vi "Read RT hardware channels.vi"(8 "error in":errorcluster, 11 "Ballard ARINC-429 Tx Execution Unit in":refnum<class "Ballard ARINC-429 Tx Scheduled Labels Execution Unit.lvclass">) -> (0 "error out":errorcluster, 2 "RT hardware channels":T1[](array[typedef]) {"labels settings for RT"."Label Timestamp Channel Data Reference" format="%.0x"; "labels settings for RT"."Word Initial Raw Value" format="%032.0f"; "labels settings for RT"."Label Disable/Trigger Channel Reference" format="%.0x"; "labels settings for RT"."parameter driver data"."Tx parameter refs" format="%.0x"; "labels settings for RT"."parameter driver data"."Rx block data refs"."Data Reference" format="%.0x"; "labels settings for RT"."SDI" format="%02b"; "labels settings for RT"."label" format="%.0o"}, 3 "Ballard ARINC-429 Tx Execution Unit out":refnum<class "Ballard ARINC-429 Tx Scheduled Labels Execution Unit.lvclass">)   [LabVIEW 2020, in "Ballard ARINC 429 Engine.lvlib" / "Implementation.lvlib" / "Ballard ARINC-429 Tx Scheduled Labels Execution Unit.lvclass"]
uses:
  Ballard ARINC-429 Tx Scheduled Labels Execution Unit.lvclass
  Shared/Label.ctl
  Encoding and Decoding/Encoding.ctl
  Encoding and Decoding/Encoding and Decoding.lvlib
  Shared/Parameter Definition.ctl
  <vilib>/NI VeriStand/Custom Device API/Data Reference.ctl
  <vilib>/NI VeriStand/Custom Device API/Custom Device API.lvlib
  <vilib>/NI VeriStand/Custom Device API/Block Data Reference.ctl
  <vilib>/NI VeriStand/Custom Device API/Custom Device Item Ref.ctl
  Shared/RT Parameters.ctl
  Shared/Transfer Type.ctl
  Shared/RT Label Settings.ctl
  Shared/RT Hardware Channel Settings.ctl
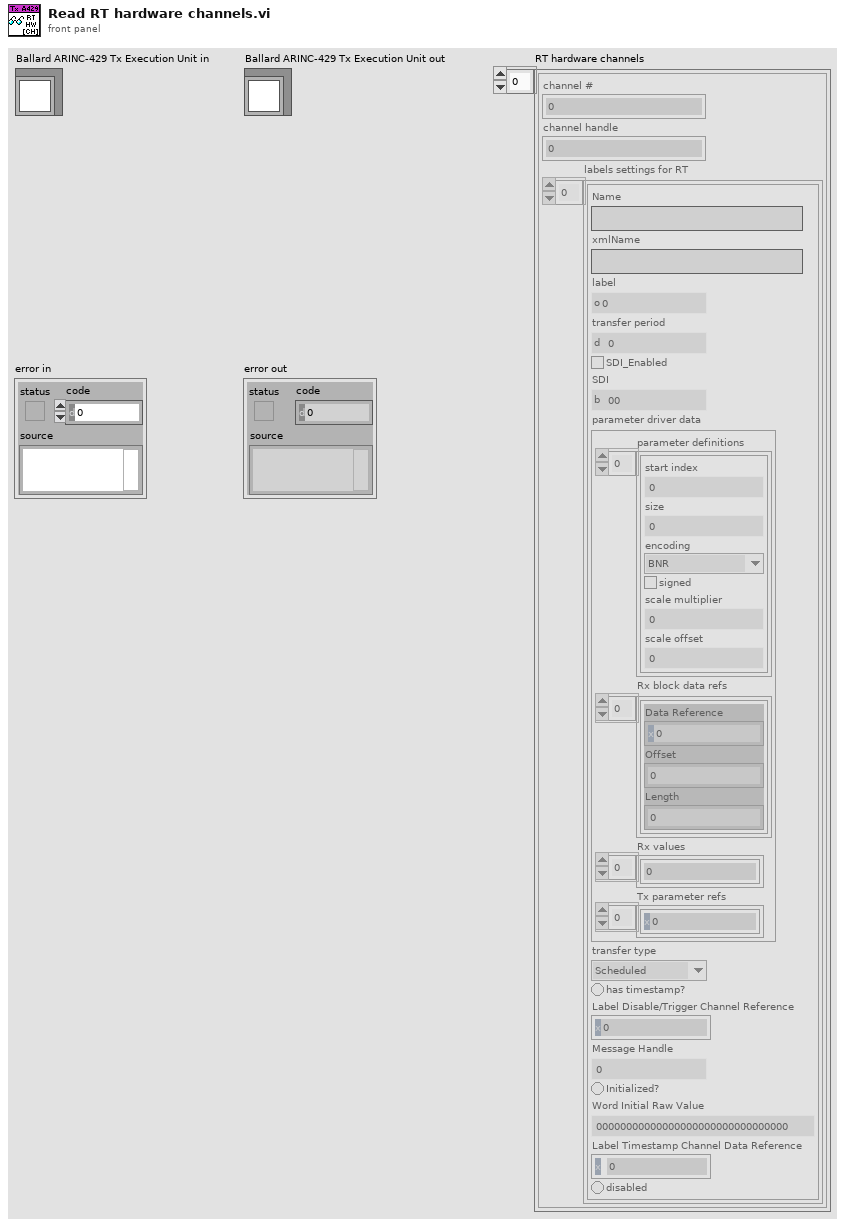
[diagram p1: front panel]
types:
  T1 = typedef "RT Hardware Channel Settings.ctl" = cluster{"channel #":u16, "channel handle":u64, "labels settings for RT":T2[]}
  T2 = typedef "RT Label Settings.ctl" = cluster{"Name":string, "xmlName":string, "label":T3, "transfer period":u32, "SDI_Enabled":bool, "SDI":u8, "parameter driver data":T4, "transfer type":T10, "has timestamp?":bool, "Label Disable/Trigger Channel Reference":T9, "Message Handle":u64, "Initialized?":bool, "Word Initial Raw Value":u32, "Label Timestamp Channel Data Reference":T8, "disabled":bool}
  T3 = typedef "Label.ctl" = u8
  T4 = typedef "RT Parameters.ctl" = cluster{"parameter definitions":T5[], "Rx block data refs":T7[], "Rx values":dbl[], "Tx parameter refs":T9[]}
  T5 = typedef "Parameter Definition.ctl" = cluster{"start index":i32, "size":i32, "encoding":T6, "signed":bool, "scale multiplier":dbl, "scale offset":dbl}
  T6 = typedef "Encoding and Decoding.lvlib/Encoding.ctl" = enum16{"BNR", "BCD", "Discrete"}
  T7 = typedef "Custom Device API.lvlib/Block Data Reference.ctl" = cluster{"Data Reference":T8, "Offset":u64, "Length":u64}
  T8 = typedef "Custom Device API.lvlib/Data Reference.ctl" = i32
  T9 = typedef "Custom Device API.lvlib/Custom Device Item Ref.ctl" = u64
  T10 = typedef "Transfer Type.ctl" = enum16{"Scheduled", "Acyclic", "Block", "Strobe"}
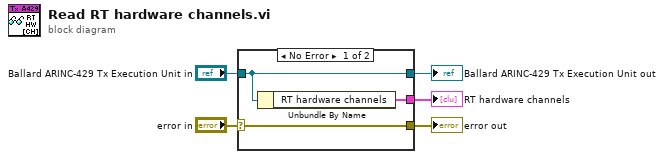
[diagram p0: block diagram]
diagram:
  n1 = case shown="No Error" "error in" {
    selector: "error in" -> [w8 w9]
    tunnel: [w8 w9] -> w4
    tunnel: [w7 w10] -> w2
    tunnel: "Ballard ARINC-429 Tx Execution Unit in" -> [w7 w10]
    tunnel: [w6 _] -> w1
    frame No Error {
      n2 = Unbundle By Name(w7) -> ("RT hardware channels"=w6:T1[])
    }
    frame Error {
    }
  }
  "error out" <- w4
  "Ballard ARINC-429 Tx Execution Unit out" <- w2
  "RT hardware channels" <- w1
